vi "Robot Global Data.vi"() -> ()   [LabVIEW 2015]
doc: "This global VI can contain as many global variables as you need. Place a control on the panel, give it a good name. To read or write to it from a VI, drag the icon to the diagram of that VI. You can also drag from the project. Click on the node to change which global you access. You shouldn't have multiple locations writing to a global or it will cause a race-condition."
uses:
  <vilib>/Rock Robotics/WPI/Camera/WPI_CameraImageSize.ctl
  <vilib>/Rock Robotics/WPI/DriverStation/WPI_DriverStationRobotMode2.ctl
panel:
  out "Right_Linear_Position":dbl
  out "Left_Linear_Position":dbl
  out "Target_Found":bool
  out "Intake_Switch":bool
  out "Auto_Aim_Running":bool
  out "Auto_Aim_Ready":bool
  in  "vision FPS":dbl
  out "Flipper_Position":dbl
  out "Gyro_Angle":dbl
  out "Right_Wheel_Encoder_Distance":dbl
  out "Left_Wheel_Encoder_Distance":dbl
  out "Linear_Actuator_Speed":dbl
  out "Enable_Manual_Shooter":bool
  out "Enable_Auto_Shooter":bool
  out "Drive_Y":dbl
  out "Drive_X":dbl
  out "Intake_Speed":dbl
  in  "Flywheel Speed Test Points":dbl[](array[numeric])
  in  "Distance Test Points":dbl[](array[numeric])
  out "Min_Distance":dbl
  out "Max_Distance":dbl
  out "Vision_Distance":dbl
  out "Sonar_Distance":dbl
  out "Centering Command":enum16{"NULL", "RIGHT", "LEFT", "CENTER"}(ring)
  out "Lower_Wheel_Suggested_Speed":dbl
  out "Lower_Flywheel_Ready":bool
  out "Upper_Flywheel_Ready":bool
  out "Upper_Wheel_Suggested_Speed":dbl
  in  "Robot Mode":T1
  in  "image size":T2=enum."320x240"
  in  "Enable Vision":bool
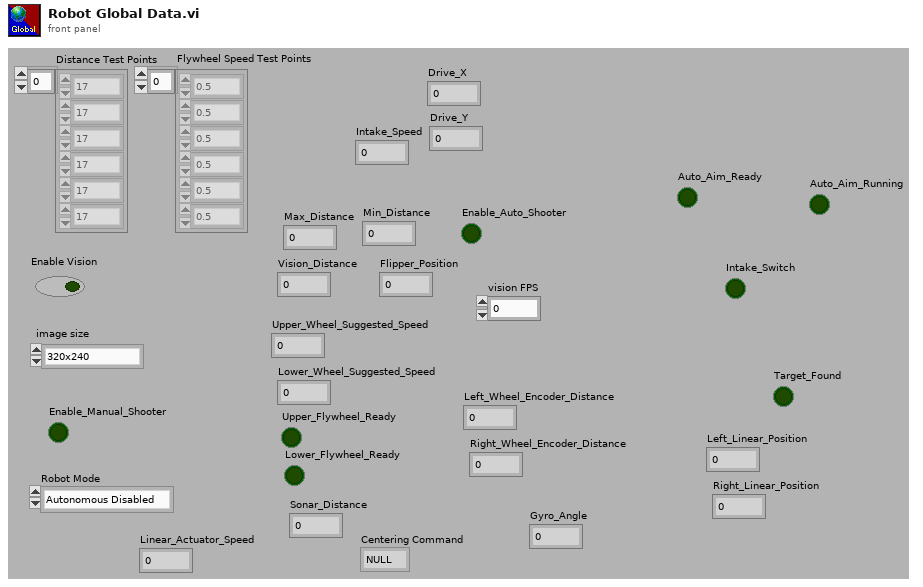
[diagram p1: front panel]
types:
  T1 = typedef "WPI_DriverStationRobotMode2.ctl" = enum16{"Autonomous Disabled", "Autonomous Enabled", "Teleop Disabled", "Teleop Enabled", "Disconnected", "Finish", "Test Disabled", "Test Enabled", "Emergency Stopped"}
  T2 = typedef "WPI_CameraImageSize.ctl" = enum16{"640x480", "320x240", "160x120", "Custom"}
diagram:
